vi "Nelson_Find_Whale.vi"(3 "error in":errorcluster, 5 "Image In":T1(plugin-control)) -> (0 "error out":errorcluster, 1 "Matches (Color Location 1)":T2(array[cluster]) {"Bounding Box"."y" format="%.2f"; "Bounding Box"."x" format="%.2f"; "Position"."y" format="%.2f"; "Position"."x" format="%.2f"; "Score" format="%.2f"; "Scale" format="%.2f"; "Angle" format="%.2f"}, 2 "Image Out":T1(plugin-control))   [LabVIEW 2014]
uses:
  <vilib>/vision/Image Controls.llb/IMAQ Image.ctl
  <vilib>/vision/NI_Vision_Development_Module.lvlib
panel:
  out "Template Image":T1(plugin-control)
  out "Image Out":T1
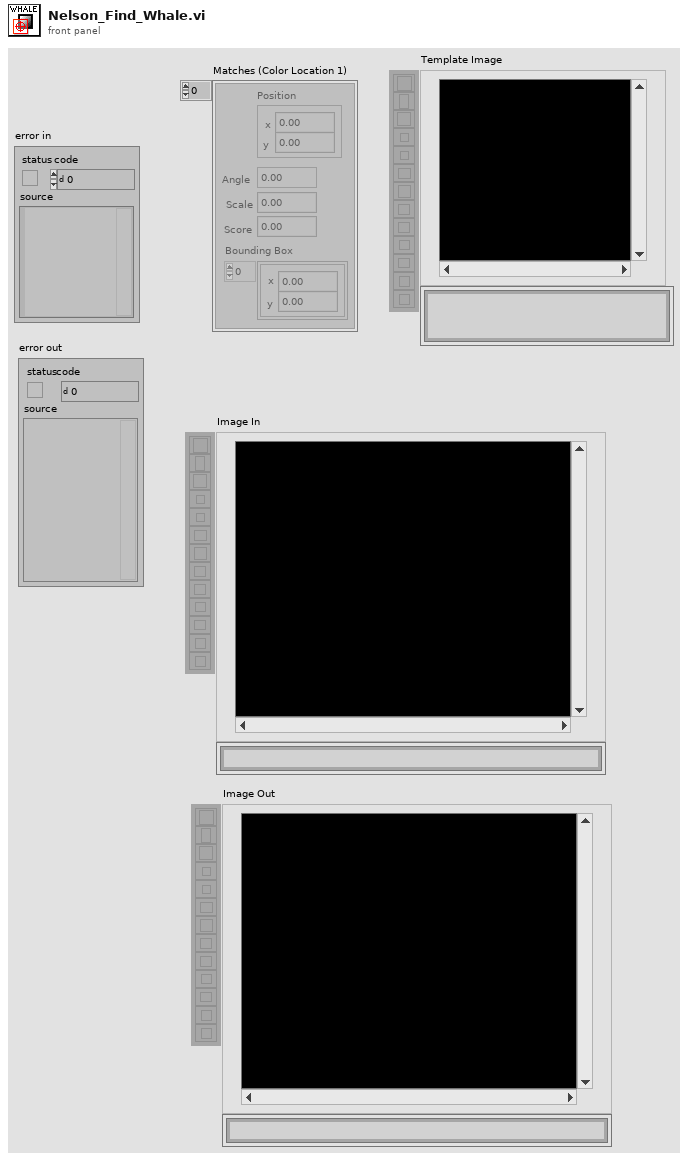
[diagram p1: front panel]
types:
  T1 = typedef "IMAQ Image.ctl" = refnum<image>
  T2 = cluster{"Position":cluster{"x":sgl, "y":sgl}, "Angle":sgl, "Scale":sgl, "Score":sgl, "Bounding Box":cluster{"x":sgl, "y":sgl}[]}[]
  T3 = typedef "Image Type" = u32
  T4 = cluster{"Global Rectangle":i32[], "Contours":cluster{"ID":enum32{"External", "Internal"}, "Type":u32, "Coordinates":i32[]}[]}
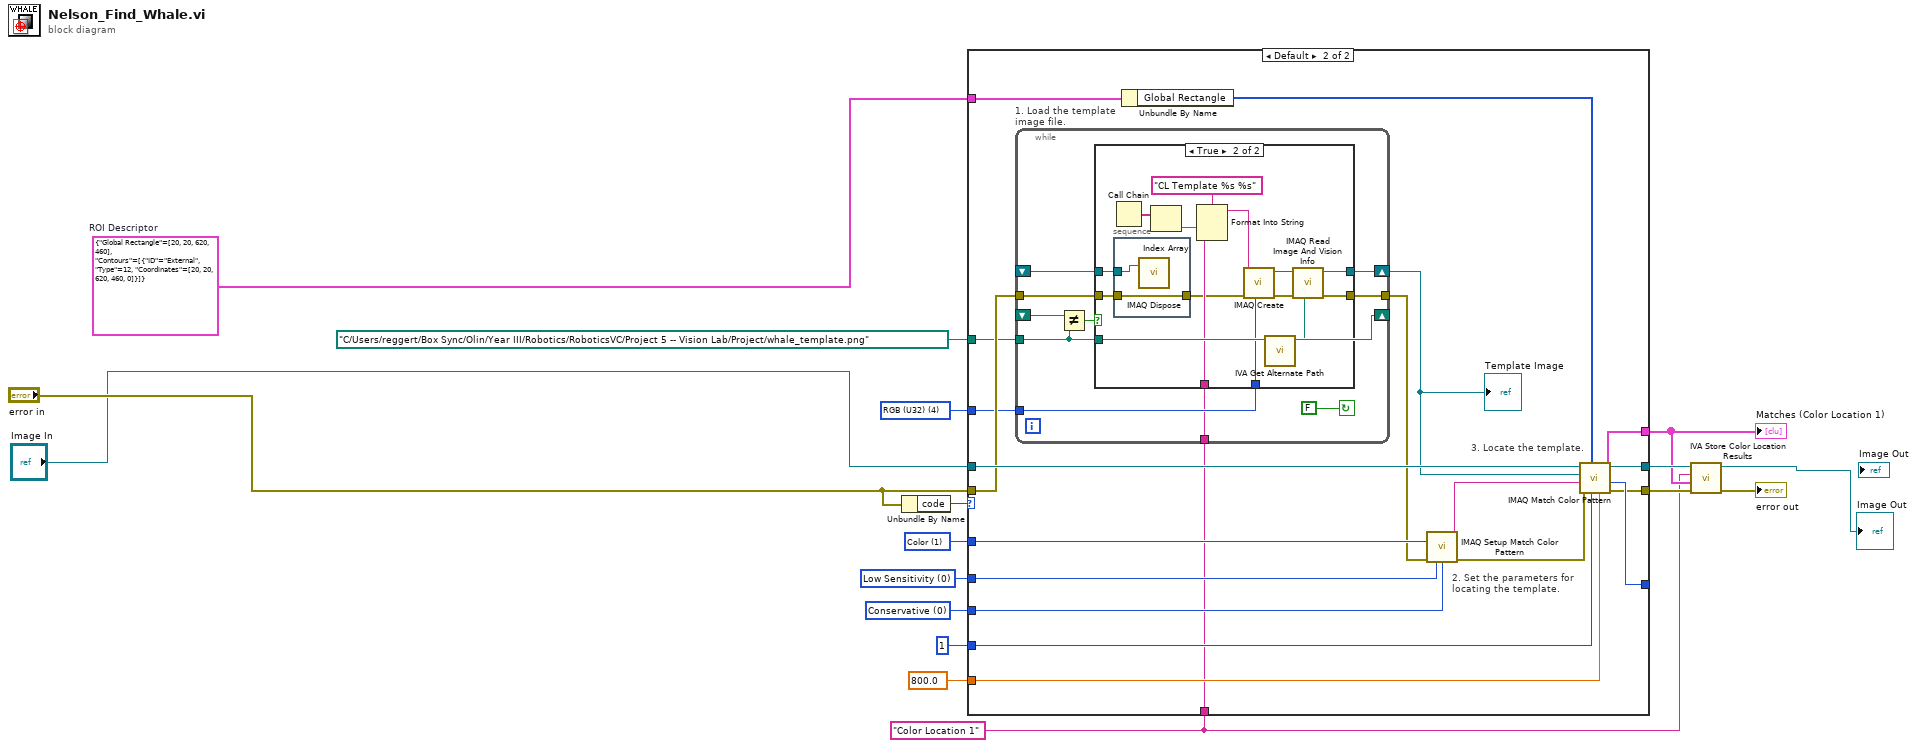
[diagram p0: block diagram]
diagram:
  w3 = "Color Location 1" ("Step Name")
  w10 = T3 4 items=["Grayscale (U8)", "Grayscale (I16)", "Grayscale (SGL)", "Complex (CSG)", "RGB (U32)", "HSL (U32)", "RGB (U64)"] ("Image Type")
  w12 = u32 0 items=["Conservative", "Balance", "Aggressive", "Very Aggressive"] ("Search Strategy")
  w13 = u32 0 items=["Low Sensitivity", "Medium Sensitivity", "High Sensitivity"] ("Color Sensitivity")
  w14 = u32 1 items=["Color and Shape", "Color", "Shape"] ("Match Feature Mode")
  w9 = T4 {"Global Rectangle"=[20, 20, 620, 460], "Contours"=[{"ID"=enum."External", "Type"=12, "Coordinates"=[20, 20, 620, 460, 0]}]}  # ROI Descriptor
  n1 = Unbundle By Name("error in") -> ("code"=w8:i32)
  n2 = case shown="Default" w8 {
    tunnel: sgl 800.0 ("Minimum Match Score") -> [_ w37]
    tunnel: 1 ("Number of Matches Requested") -> [_ w36]
    tunnel: [_ w35] -> _
    tunnel: w14 -> [_ w34]
    tunnel: w13 -> [_ w33]
    tunnel: w12 -> [_ w32]
    tunnel: path "C:/Users/reggert/Box Sync/Olin/Year III/Robotics/RoboticsVC/Project 5 -- Vision Lab/Project/whale_template.png" ("File Path") -> [_ w24]
    tunnel: w10 -> [_ w23]
    tunnel: "error in" -> [_ w25]
    tunnel: w9 -> [_ w29]
    tunnel: [_ w27] -> w4
    tunnel: "Image In" -> [w18 w26]
    tunnel: [w18 w26] -> w5
    tunnel: [_ w21] -> w6
    tunnel: w3 -> [_ w20]
    frame -1074396199, -1074396198 {
      # "Discard Coordinate System Error"
    }
    frame Default {
      # "3. Locate the template."
      # "2. Set the parameters for\nlocating the template."
      n3 = while "1. Load the template image file." {
        shift-right: [w47] -> w19
        shift-left: _ -> [w46]
        tunnel: [w44] -> w22
        tunnel: w25 -> [w43]
        tunnel: w24 -> [w38]
        tunnel: w23 -> [w42]
        tunnel: w20 -> [w41]
        shift-right: [w38] -> _
        shift-left: _ -> [w40]
        stop <- FALSE continue-if-true
        n4 = Not Equal?(x=w40, y=w38) -> (x != y?=w39:bool)
        n5 = case shown="True" w39 {
          tunnel: [w49 w62] -> w47
          tunnel: w46 -> [w49 w54]
          tunnel: [w48 w59] -> w44
          tunnel: w43 -> [w48 w53]
          tunnel: w42 -> [_ w58]
          tunnel: w41 -> [_ w55]
          tunnel: w38 -> [_ w51]
          frame False {
          }
          frame True {
            n6 = Call Chain() -> (call chain=w57:string[])
            n7 = stacked-sequence {
              tunnel: w54 -> [w66]
              tunnel: w53 -> [w65]
              tunnel: [w65] -> w52
              frame #0 {
                n8 = call "IMAQ Dispose"("Image"=w66) -> ()  [unwired: 2 in, 4 out]
              }
            }
            n9 = Index Array(array=w57) -> (element=w56:string)  [unwired: 1 in]
            n10 = Format Into String(format string="CL Template %s %s" ("Image Name"), w56, w55) -> (resulting string=w64:string)  [unwired: 2 in, 1 out]
            n11 = call "IMAQ Create"("Image Name"=w64, "Image Type"=w58, "error in (no error)"=w52) -> ("New Image"=w61:T1, "error out"=w60:errorcluster)  [unwired: 1 in, 1 out]
            n12 = call <vilib>:"IVA Get Alternate Path.vi"("Path In"=w51) -> ("Path Out"=w50:path)  [unwired: 10 out]
            n13 = call "IMAQ Read Image And Vision Info"("File Path"=w50, "error in (no error)"=w60, "Image"=w61) -> ("error out"=w59:errorcluster, "Image Out"=w62:T1)  [unwired: 1 in, 6 out]
          }
        }
      }
      "Template Image" <- w19
      n14 = Unbundle By Name(w29) -> ("Global Rectangle"=w28:i32[])
      n15 = call "IMAQ Setup Match Color Pattern"("Match Feature Mode"=w34, "error in (no error)"=w22, "Color Sensitivity"=w33, "Search Strategy"=w32) -> ("Match Color Pattern Setup Data"=w31:string, "error out"=w30:errorcluster)  [unwired: 5 in, 5 out]
      n16 = call "IMAQ Match Color Pattern"("Minimum Match Score"=w37, "Number of Matches Requested"=w36, "Optional Rectangle"=w28, "error in (no error)"=w30, "Match Color Pattern Setup Data"=w31, "Template Image"=w19, "Image"=w26) -> ("error out"=w21:errorcluster, "Number of Matches"=w35:i32, "Matches"=w27:T2)  [unwired: 2 out]
    }
  }
  "Matches (Color Location 1)" <- w4
  n17 = call <vilib>:"IVA Store Color Location Results.vi"("error in (no error)"=w6, "Matches"=w4, "Step Name"=w3, "Image in"=w5) -> ("error out"=→"error out":errorcluster, "Image dup"=→"Image Out":T1)  [unwired: 6 out]
